vi "防死机.vi"(5 "精度":dbl, 6 "起始值":dbl, 7 "实时值":dbl, 8 "序":i32, 10 "CMD":string, 11 "IN":refnum<visa-resource-name>) -> (3 "OUT":refnum<visa-resource-name>)   [LabVIEW 2016]
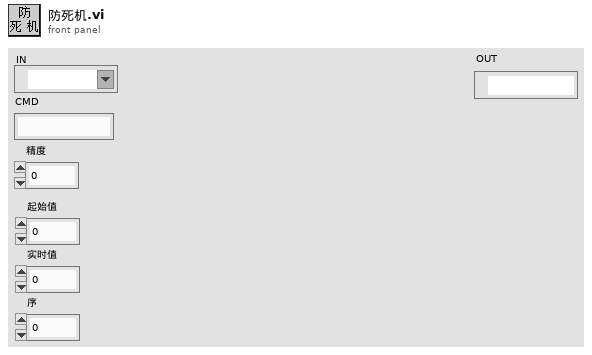
[diagram p1: front panel]
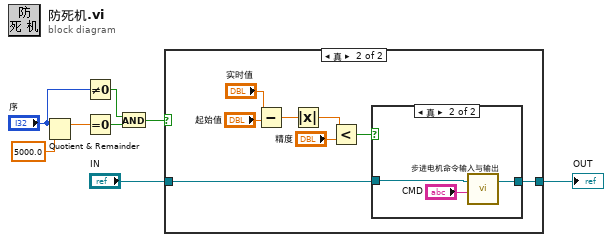
[diagram p0: block diagram]
diagram:
  n1 = Quotient & Remainder(x="序", y=5000.0) -> (x-y*floor(x/y)=w3:dbl)  [unwired: 1 out]
  n2 = Not Equal To 0?(x="序") -> (x != 0?=w2:bool)
  n3 = Equal To 0?(x=w3) -> (x = 0?=w4:bool)
  n4 = And(x=w2, y=w4) -> (x .and. y?=w5:bool)
  n5 = case shown="真" w5 {
    tunnel: "IN" -> [w9 w11]
    tunnel: [w9 w10] -> w7
    frame False {
    }
    frame True {
      n6 = Subtract(x="实时值", y="起始值") -> (x-y=w14:dbl)
      n7 = Absolute Value(x=w14) -> (abs(x)=w15:dbl)
      n8 = Less?(x=w15, y="精度") -> (x < y?=w17:bool)
      n9 = case shown="真" w17 {
        tunnel: w11 -> [w18 w20]
        tunnel: [w18 w19] -> w10
        frame False {
        }
        frame True {
          n10 = call "步进电机命令输入与输出.vi"("输入字符串"="CMD", "串口通信端口"=w20) -> ("VISA资源名称输出"=w19:refnum<visa-resource-name>)  [unwired: 1 out]
        }
      }
    }
  }
  "OUT" <- w7
